vi "Server.vi"() -> ()   [LabVIEW 2022 SP3]
panel:
  out "data out":string
  out "error out":errorcluster
  out "time string":string
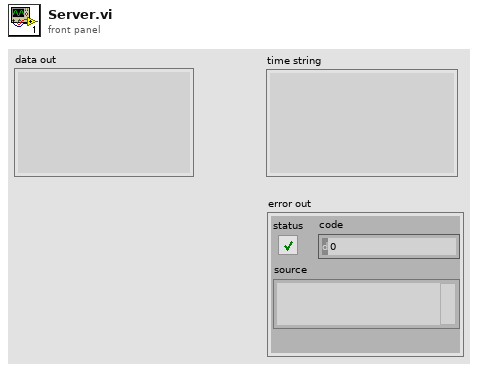
[diagram p1: front panel]
types:
  T1 = enum16{"Standard", "Buffered", "CRLF", "Immediate"}
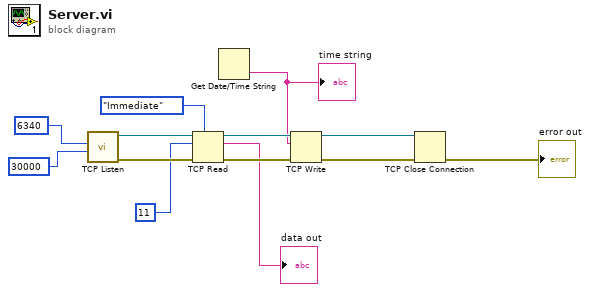
[diagram p0: block diagram]
diagram:
  n1 = call <vilib>:"TCP Listen.vi"("timeout ms (wait forever: -1)"=30000, "port"=u16 6340) -> ("error out"=w12:errorcluster, "connection ID"=w13:refnum<k5>)  [unwired: 5 in, 3 out]
  n2 = TCP Read(connection ID=w13, bytes to read=11, error in (no error)=w12, 7:T1."Immediate" ("mode (standard)")) -> (connection ID out=w11:refnum<k5>, data out=→"data out":string, error out=w10:errorcluster)  [unwired: 1 in]
  n3 = Get Date/Time String() -> (time string=w7:string)  [unwired: 3 in, 1 out]
  "time string" <- w7
  n4 = TCP Write(connection ID=w11, data in=w7, error in (no error)=w10) -> (connection ID out=w9:refnum<k5>, error out=w8:errorcluster)  [unwired: 1 in, 1 out]
  n5 = TCP Close Connection(connection ID=w9, error in (no error)=w8) -> (error out=→"error out":errorcluster)  [unwired: 1 in, 1 out]
